vi "Save1 INI.vi"(9 "parameter Input":T1, 11 "名称或相对路径":string="UserDefine.ini") -> ()   [LabVIEW 2011]
uses:
  Global System.vi
  <vilib>/Utility/config.llb/NI_LVConfig.lvlib
panel:
  in  "Keys":string[](array[string])=["StrVel", "MaxVel", "MarkPs", "Step1_S", "Step1_E", "Step2_S", "Step2_E", "Step3_S", "Step3_E", "Step4_S", "Step4_E"]
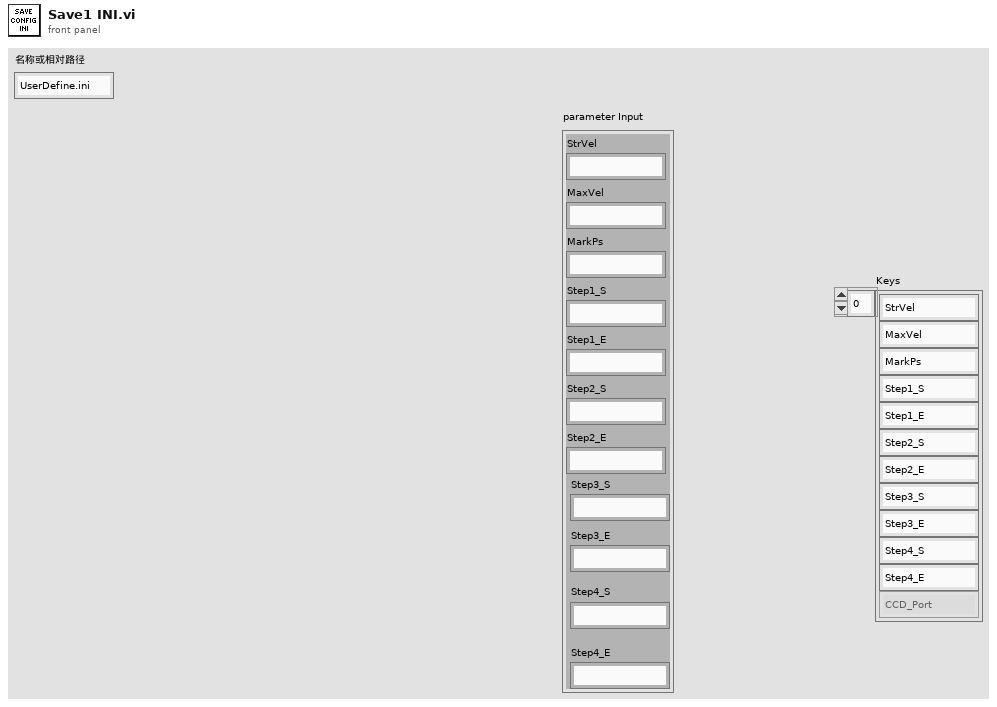
[diagram p1: front panel]
types:
  T1 = cluster{"StrVel":string, "MaxVel":string, "MarkPs":string, "Step1_S":string, "Step1_E":string, "Step2_S":string, "Step2_E":string, "Step3_S":string, "Step3_E":string, "Step4_S":string, "Step4_E":string}
  T2 = cluster{"PLC窗口名称":refnum<visa-resource-name>, "CCD_TcpName":string, "CCD_Port":string, "ShopFloor":string, "SW Rev":string, "Reserved":string, "Active Barcode":string, "Active PDCA":string, "Build Date":string, "SW Updated":string, "Total Life Cycles":string, "Total Life Rejects":string}
  T3 = typedef "NI_LVConfig.lvlib/Config Data RefNum.ctl" = refnum<k1>
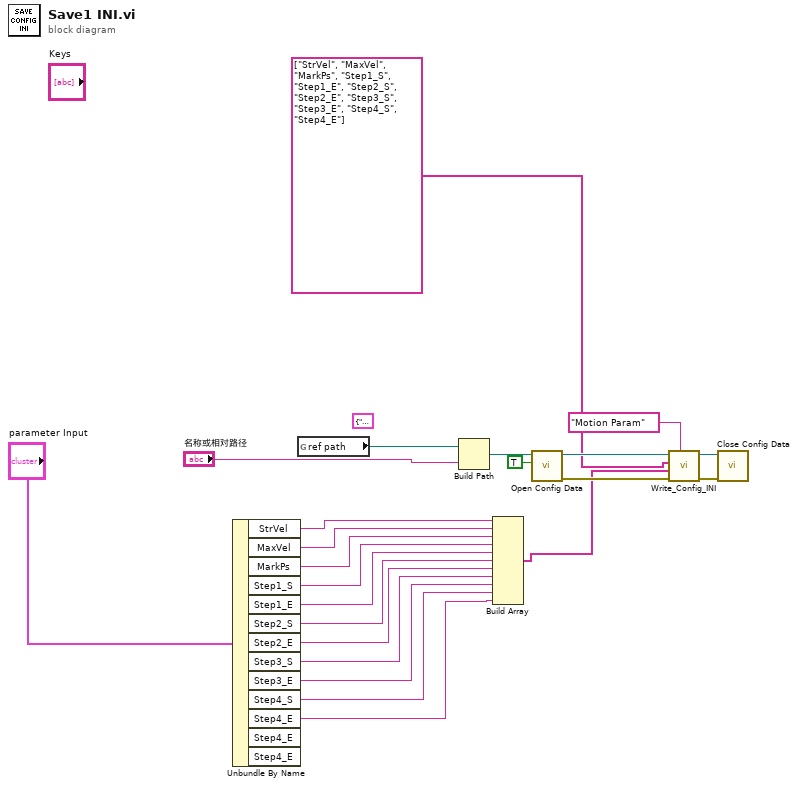
[diagram p0: block diagram]
diagram:
  (unwired) T2 {"PLC窗口名称"="", "CCD_TcpName"="", "CCD_Port"="", "ShopFloor"="", "SW Rev"="", "Reserved"="", "Active Barcode"="", "Active PDCA"="", "Build Date"="", "SW Updated"="", "Total Life Cycles"="", "Total Life Rejects"=""} ("parameter Input 2")
  n1 = Unbundle By Name("parameter Input") -> ("StrVel"=w12:string, "MaxVel"=w11:string, "MarkPs"=w10:string, "Step1_S"=w9:string, "Step1_E"=w8:string, "Step2_S"=w7:string, "Step2_E"=w6:string, "Step3_S"=w4:string, "Step3_E"=w3:string, "Step4_S"=w2:string, "Step4_E"=w1:string)  [unwired: 2 out]
  n2 = global read "Global System.vi" "ref path"() -> (w23:path)
  n3 = Build Path(base path=w23, name or relative path="名称或相对路径") -> (appended path=w20:path)
  n4 = Build Array(w12, w11, w10, w9, w8, w7, w6, w4, w3, w2, w1) -> (w5:string[])
  n5 = call <vilib>:"Open Config Data.vi"("create file if necessary (T)"=TRUE, "configuration file path"=w20) -> ("error out"=w18:errorcluster, "refnum"=w19:T3)  [unwired: 7 in, 1 out]
  n6 = call "Write_Config_INI.vi"("section"="Motion Param", "error in (no error)"=w18, "Inputs"=w5, "Keys"=string[] ["StrVel", "MaxVel", "MarkPs", "Step1_S", "Step1_E", "Step2_S", "Step2_E", "Step3_S", "Step3_E", "Step4_S", "Step4_E"], "refnum"=w19) -> ("error out"=w15:errorcluster, "refnum 2"=w16:T3)  [unwired: 5 in]
  n7 = call <vilib>:"Close Config Data.vi"("error in (no error)"=w15, "refnum"=w16) -> ()  [unwired: 8 in, 2 out]
